vi "Test.vi"() -> ()   [LabVIEW 2021, in "BNT_DSCXtGraph.lvlib"]
uses:
  BNT_DSCXtGraph.lvlib
  <vilib>/lvdsc/historical/Read Traces (Numeric).vi
  <vilib>/lvdsc/NI_DSC.lvlib
panel:
  out "max array size":i32
  out "min array size":i32
  out "min(x,y)":timestamp
  out "max(x,y)":timestamp
  out "historical traces":T1(array[cluster]) {"data" format="%0.6f"; "timestamps" format="%<%X\n%x>T"}
  out "XY Graph":T1(graph)
  out "quality":i32[][](array[numeric])
  in  "options":T2={"interpolate data (F)"=FALSE, "extrapolate to now (F)"=FALSE, "remove data breaks (F)"=FALSE, "interpolation interval (1 s)"=1.0, "maintain trending info (T)"=TRUE} {"interpolation interval (1 s)" min=0.0 format="%0.2f"}
  in  "time interval":T3 {"stop timestamp (now)" format="%<%X\n%x>T"; "start timestamp" format="%<%X\n%x>T"}
  in  "max points per trace (all)":i32=-1
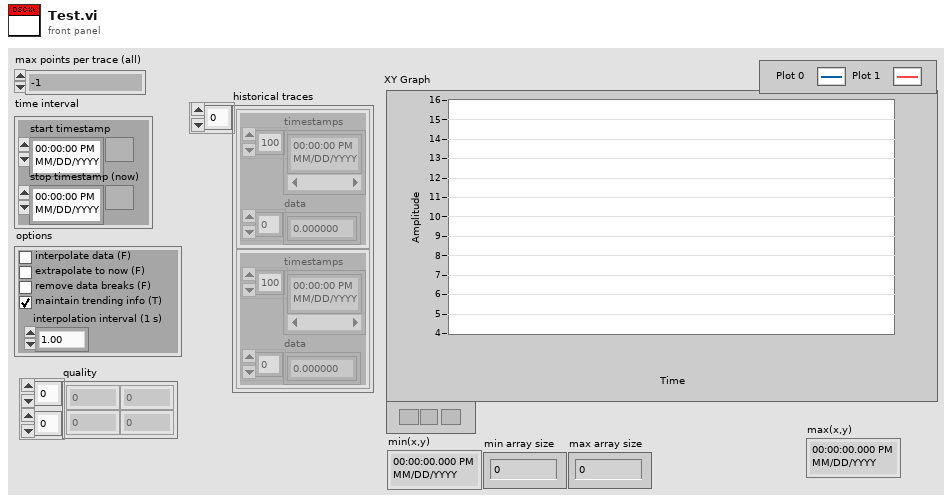
[diagram p1: front panel]
types:
  T1 = cluster{"timestamps":timestamp[], "data":dbl[]}[]
  T2 = cluster{"interpolate data (F)":bool, "extrapolate to now (F)":bool, "remove data breaks (F)":bool, "interpolation interval (1 s)":dbl, "maintain trending info (T)":bool}
  T3 = cluster{"start timestamp":timestamp, "stop timestamp (now)":timestamp}
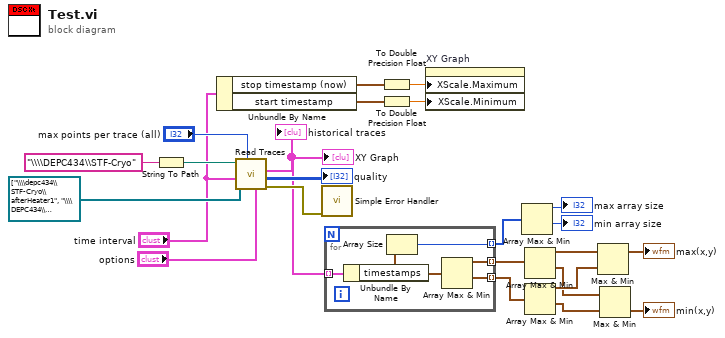
[diagram p0: block diagram]
diagram:
  n1 = String To Path(string="\\\\DEPC434\\STF-Cryo") -> (path=w24:path)
  n2 = Unbundle By Name("time interval") -> ("stop timestamp (now)"=w2:timestamp, "start timestamp"=w1:timestamp)
  n3 = call-poly <vilib>:"Read Traces.vi"("options"="options", "max points per trace (all)"="max points per trace (all)", "time interval"="time interval", "trace names"=refnum<k21>[] ["\\\\depc434\\STF-Cryo\\afterHeater1", "\\\\DEPC434\\STF-Cryo\\afterHeater2"], "database URL"=w24) -> ("error out"=w19:errorcluster, "quality"=→"quality":i32[][], "historical traces"=w6:T1)  [unwired: 3 in, 1 out]
  "historical traces" <- w6
  "XY Graph" <- w6
  n4 = call <vilib>:"Simple Error Handler.vi"("error in (no error)"=w19) -> ()  [unwired: 4 in, 5 out]
  n5 = for {
    tunnel: w6 -> [w29] mode=indexing
    tunnel: [w28] -> w17 mode=indexing
    tunnel: [w27] -> w16 mode=indexing
    tunnel: [w25] -> w9 mode=indexing
    n6 = Unbundle By Name(w29) -> ("timestamps"=w26:timestamp[])
    n7 = Array Size(array=w26) -> (size(s)=w25:i32)
    n8 = Array Max & Min(array=w26) -> (max value=w28:timestamp, min value=w27:timestamp)  [unwired: 2 out]
  }
  n9 = To Double Precision Float(number=w2) -> (double precision float=w4:dbl)
  n10 = To Double Precision Float(number=w1) -> (double precision float=w5:dbl)
  n11 = property on="XY Graph" class="XYGraph (strict)"("XScale.Maximum"=w4, "XScale.Minimum"=w5) -> ()  [unwired: 2 in, 2 out]
  n12 = Array Max & Min(array=w9) -> (max value=→"max array size":i32, min value=→"min array size":i32)  [unwired: 2 out]
  n13 = Array Max & Min(array=w17) -> (max value=w14:timestamp, min value=w13:timestamp)  [unwired: 2 out]
  n14 = Array Max & Min(array=w16) -> (max value=w15:timestamp, min value=w12:timestamp)  [unwired: 2 out]
  n15 = Max & Min(x=w14, y=w15) -> (max(x,y)=→"max(x,y)":timestamp)  [unwired: 1 out]
  n16 = Max & Min(x=w13, y=w12) -> (min(x,y)=→"min(x,y)":timestamp)  [unwired: 1 out]
